vi "Keithley 6517 Relative Measurement.vi"() -> ()   [LabVIEW 2016]
doc: "Configures and exexutes a Rel'd measurement for model 6514. \n\n<B>Note:</B>\nThis examples is ONLY for <B>model 6514."
uses:
  <instrlib>/Keithley 6517/Keithley 6517.lvlib
panel:
  in  "Timeout (10000 ms)":u32=10000
  in  "Arm Count (1)":i32=1
  in  "VISA resource name":refnum<visa-resource-name>
  out "Rel'd Measurement Data":dbl[][](array[numeric])
  in  "Limit Test Source (0: SENSE)":u16(ring) items=["Measurements (SENSE)", "Math Calculations (CALC1)"]
  in  "Rel Value (0)":dbl=1.0
  in  "Measurement Function (0: Voltage)":i32(ring) items=["Voltage", "Current", "Resistance", "Charge"]
  # "(c) 2016-2017 National Instruments.  ALL RIGHTS RESERVED."
  # "Note: This Example is ONLY compatible with model 6514."
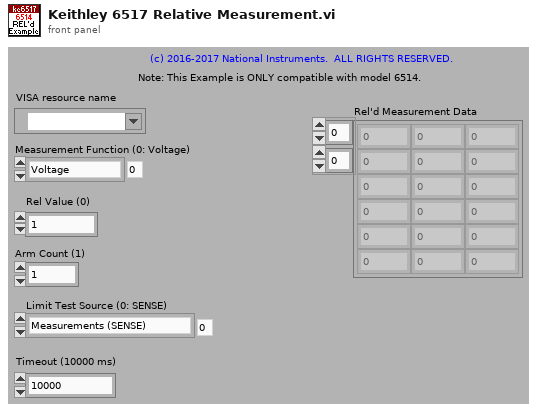
[diagram p1: front panel]
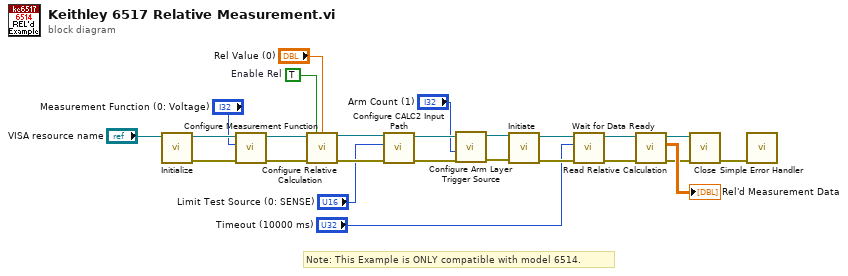
[diagram p0: block diagram]
diagram:
  w17 = TRUE  # Enable Rel
  # "Note: This Example is ONLY compatible with model 6514."
  n1 = call <instrlib>:"Initialize.vi"("VISA resource name"="VISA resource name") -> ("error out"=w25:errorcluster, "VISA resource name out"=w24:refnum<visa-resource-name>)  [unwired: 9 in]
  n2 = call <instrlib>:"Configure Measurement Function.vi"("error in (no error)"=w25, "Measurement Function (0: Voltage)"="Measurement Function (0: Voltage)", "VISA resource name"=w24) -> ("error out"=w23:errorcluster, "VISA resource name out"=w22:refnum<visa-resource-name>)  [unwired: 7 in]
  n3 = call <instrlib>:"Configure Relative Calculation.vi"("VISA resource name"=w22, "Enable Rel (F: Disable)"=w17, "Rel Value (0)"="Rel Value (0)", "error in (no error)"=w23) -> ("VISA resource name out"=w20:refnum<visa-resource-name>, "error out"=w21:errorcluster)  [unwired: 10 in]
  n4 = call <instrlib>:"Configure CALC2 Input Path.vi"("error in (no error)"=w21, "Limit Test Source (0: SENSE)"="Limit Test Source (0: SENSE)", "VISA resource name"=w20) -> ("error out"=w13:errorcluster, "VISA resource name out"=w10:refnum<visa-resource-name>)  [unwired: 7 in]
  n5 = call <instrlib>:"Configure Arm Layer Trigger Source.vi"("error in (no error)"=w13, "Arm Count (1)"="Arm Count (1)", "VISA resource name"=w10) -> ("error out"=w12:errorcluster, "VISA resource name out"=w11:refnum<visa-resource-name>)  [unwired: 7 in]
  n6 = call <instrlib>:"Initiate.vi"("error in (no error)"=w12, "VISA resource name"=w11) -> ("error out"=w8:errorcluster, "VISA resource name out"=w7:refnum<visa-resource-name>)  [unwired: 8 in]
  n7 = call <instrlib>:"Wait for Data Ready.vi"("error in (no error)"=w8, "Timeout (10000 ms)"="Timeout (10000 ms)", "VISA resource name"=w7) -> ("error out"=w5:errorcluster, "VISA resource name out"=w6:refnum<visa-resource-name>)  [unwired: 7 in]
  n8 = call <instrlib>:"Read Relative Calculation.vi"("error in (no error)"=w5, "VISA resource name"=w6) -> ("error out"=w3:errorcluster, "Rel'd Measurement Data"=→"Rel'd Measurement Data":dbl[][], "VISA resource name out"=w2:refnum<visa-resource-name>)  [unwired: 7 in]
  n9 = call <instrlib>:"Close.vi"("error in (no error)"=w3, "VISA resource name"=w2) -> ("error out"=w1:errorcluster)  [unwired: 9 in]
  n10 = call <vilib>:"Simple Error Handler.vi"("error in (no error)"=w1) -> ()  [unwired: 4 in, 5 out]
